vi "APT_Joystick.vi"() -> ()   [LabVIEW 2015]
uses:
  <vilib>/Utility/inputDevices.llb/joystickAcquire.vi
  Global Variable/GV_Lock State.vi
  Global Variable/GV_Z axis.vi
  <vilib>/Utility/inputDevices.llb/closeJoystick.vi
panel:
  out "Lock State":dbl=18.0
  out "lock":bool
  in  "error in (no error)":errorcluster caption="错误输入（无错误）"
  in  "MG17Motor Y":refnum<k7>(container)
  in  "选项卡控件":enum32{"APT Controller", "Parameters"}(tab)
  in  "Absolute y":dbl
  in  "Stop Device":bool
  in  "y Down":bool
  in  "y Up":bool
  out "y lock":bool
  out "x lock":bool
  in  "Joystick Onoff":bool=TRUE
  in  "HWSerialNum Y":i32=26000520
  in  "Stop":bool
  in  "Home X":bool
  in  "Rel. Pos X":dbl=0.01 min=-10.0 max=360.0 format="%.4f"
  in  "Deviece Joystick":i32=5
  out "Display X":dbl(knob)=6.2977495193481445 scale=0.0..25.0
  out "Initial X":bool=TRUE
  out "Initial Y":bool=TRUE
  out "Display Y":dbl(knob)=20.590396881103516 scale=0.0..25.0
  in  "Home Y":bool
  in  "Rel. Pos Y":dbl=0.01 min=-10.0 max=360.0 format="%.4f"
  in  "HWSerialNum X":i32=26000634
  in  "x Down":bool
  in  "x Up":bool
  in  "Absolute x":dbl
  out "操纵杆信息":T1(array[cluster])=[{"axes total"=5, "buttons total"=10, "pov total"=1, "device name"="Controller (XBOX One For Windows)"}, {"axes total"=1, "buttons total"=1, "pov total"=0, "device name"="USB Keyboard"}, {"axes total"=0, "buttons total"=3, "pov total"=0, "device name"="USB Keyboard"}, {"axes total"=0, "buttons total"=21, "pov total"=0, "device name"="USB Keyboard"}]
  out "X axis":i32=797
  out "Y axis":i32=796
  out "Z axis":i32
  out "Y axis rotation":i32=-1813
  out "Axis Info":T2={"X axis"=797, "Y axis"=796, "Z axis"=0, "X axis rotation"=1154, "Y axis rotation"=-1813, "Z axis rotation"=0, "U axis"=0, "V axis"=0}
  out "按键信息":T3
  in  "下限":dbl
  in  "上限":dbl=25.0
  out "方向信息":T4={"pov 1"=-1, "pov 2"=-1, "pov 3"=-1, "pov 4"=-1}
  in  "MG17Motor X":refnum<k7>(container)
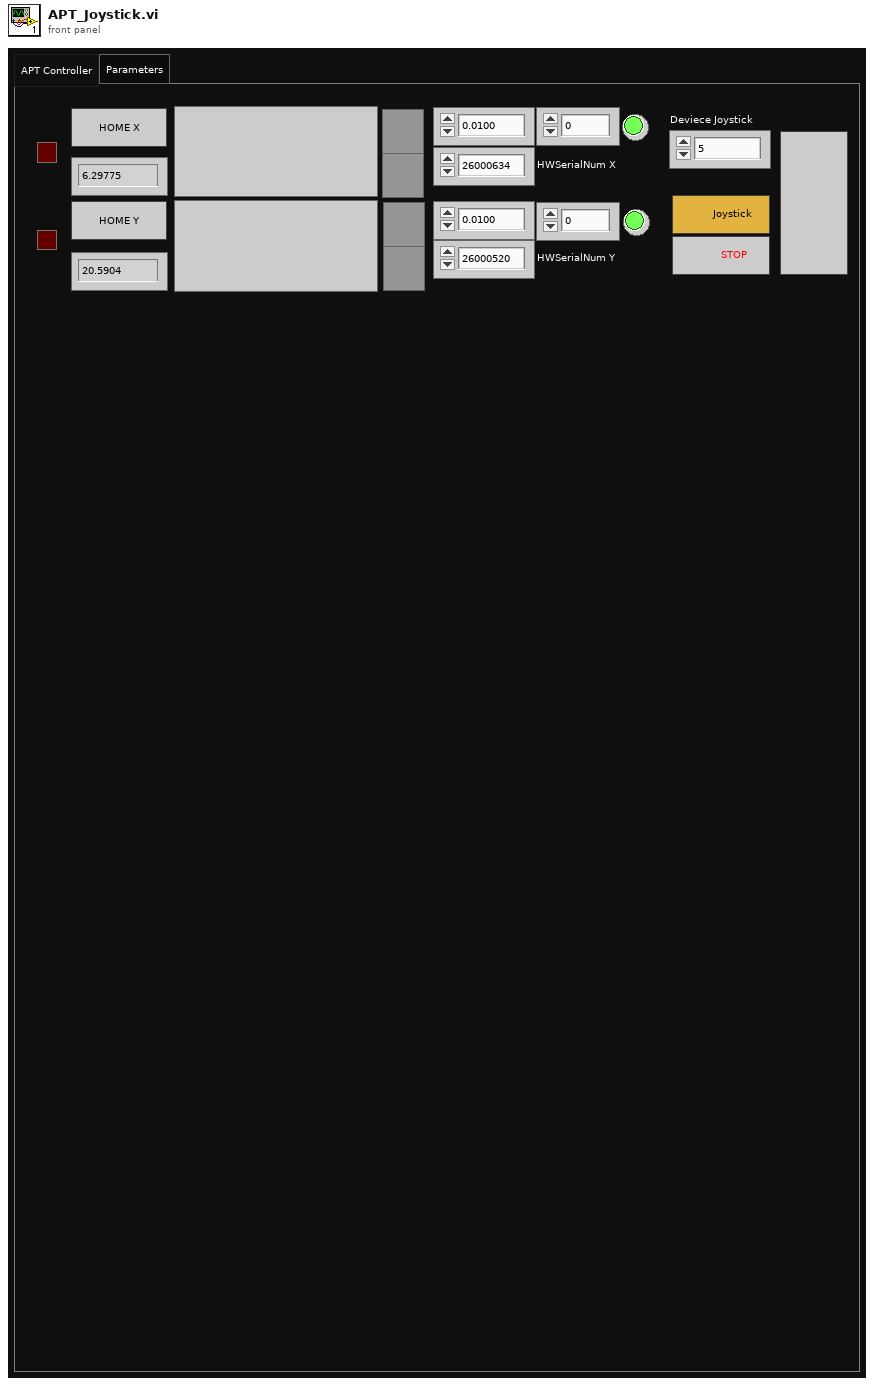
[diagram p1: front panel]
types:
  T1 = cluster{"axes total":u32, "buttons total":u32, "pov total":u32, "device name":string}[]
  T2 = cluster{"X axis":i32, "Y axis":i32, "Z axis":i32, "X axis rotation":i32, "Y axis rotation":i32, "Z axis rotation":i32, "U axis":i32, "V axis":i32}
  T3 = cluster{"button 1":bool, "button 2":bool, "button 3":bool, "button 4":bool, "button 5":bool, "button 6":bool, "button 7":bool, "button 8":bool, "button 9":bool, "button 10":bool, "button 11":bool, "button 12":bool, "button 13":bool, "button 14":bool, "button 15":bool, "button 16":bool, "button 17":bool, "button 18":bool, "button 19":bool, "button 20":bool, "button 21":bool, "button 22":bool, "button 23":bool, "button 24":bool, "button 25":bool, "button 26":bool, "button 27":bool, "button 28":bool, "button 29":bool, "button 30":bool, "button 31":bool, "button 32":bool}
  T4 = cluster{"pov 1":i32, "pov 2":i32, "pov 3":i32, "pov 4":i32}
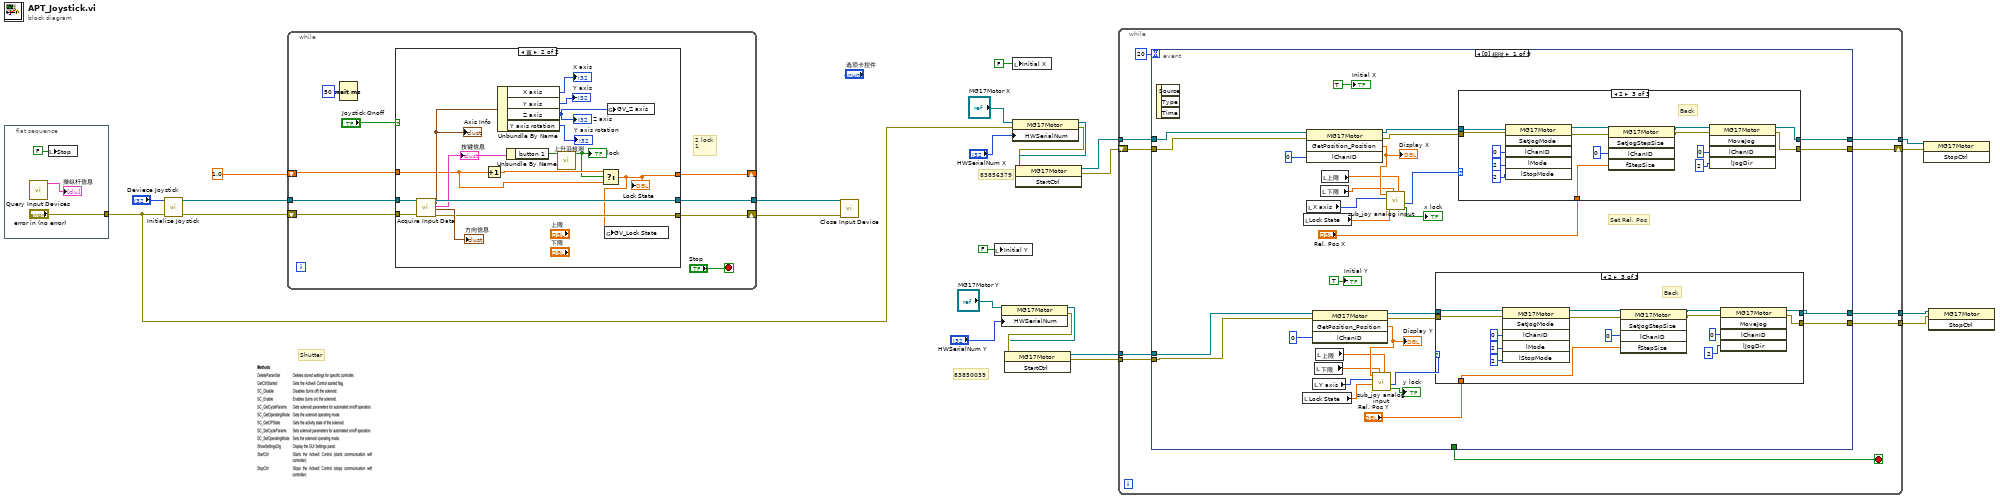
[diagram p0: block diagram]
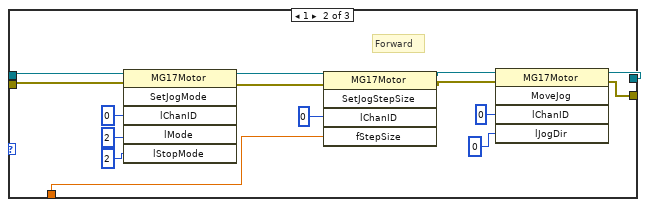
[diagram p3: hidden frame]
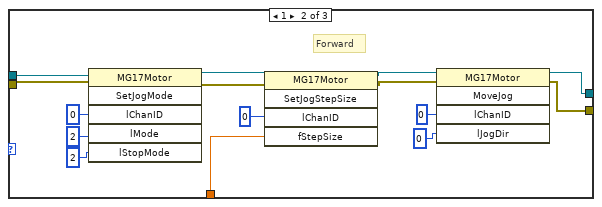
[diagram p5: hidden frame]
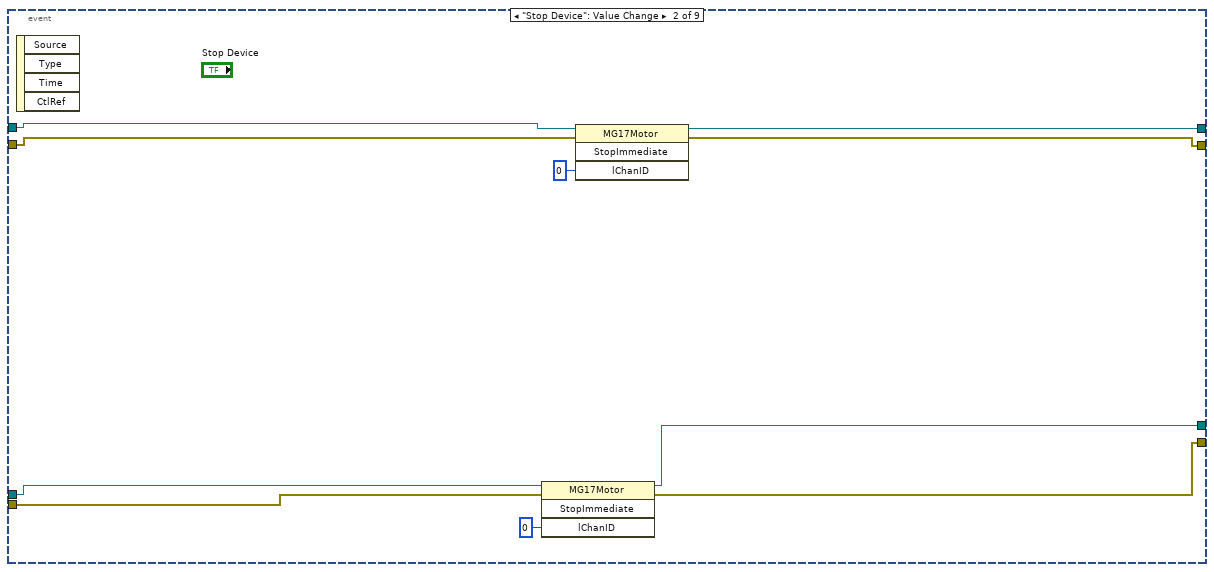
[diagram p6: hidden frame]
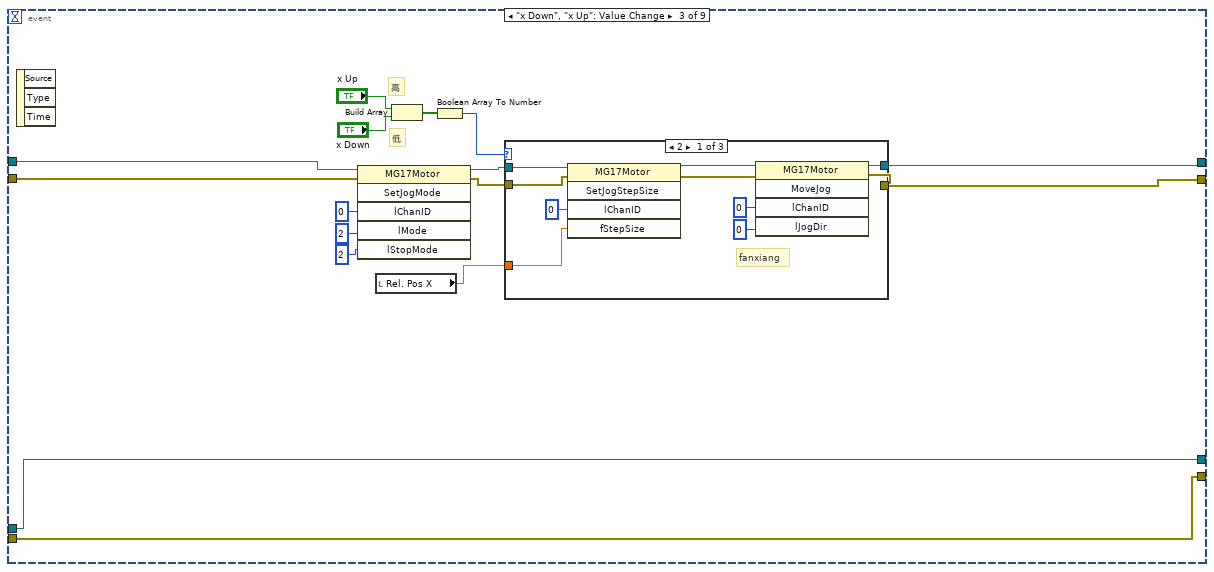
[diagram p7: hidden frame]
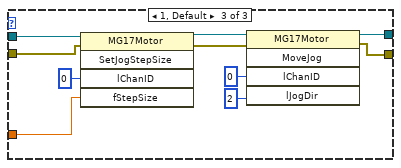
[diagram p9: hidden frame]
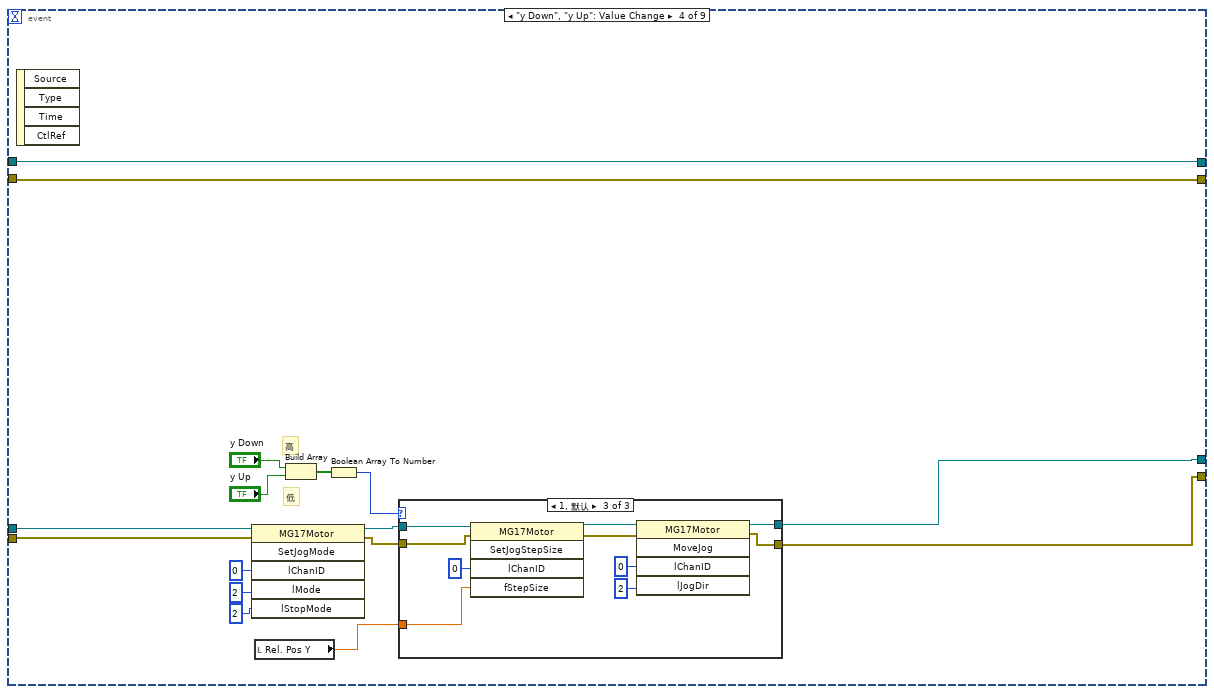
[diagram p10: hidden frame]
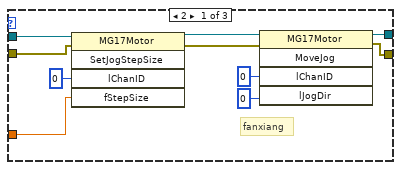
[diagram p11: hidden frame]
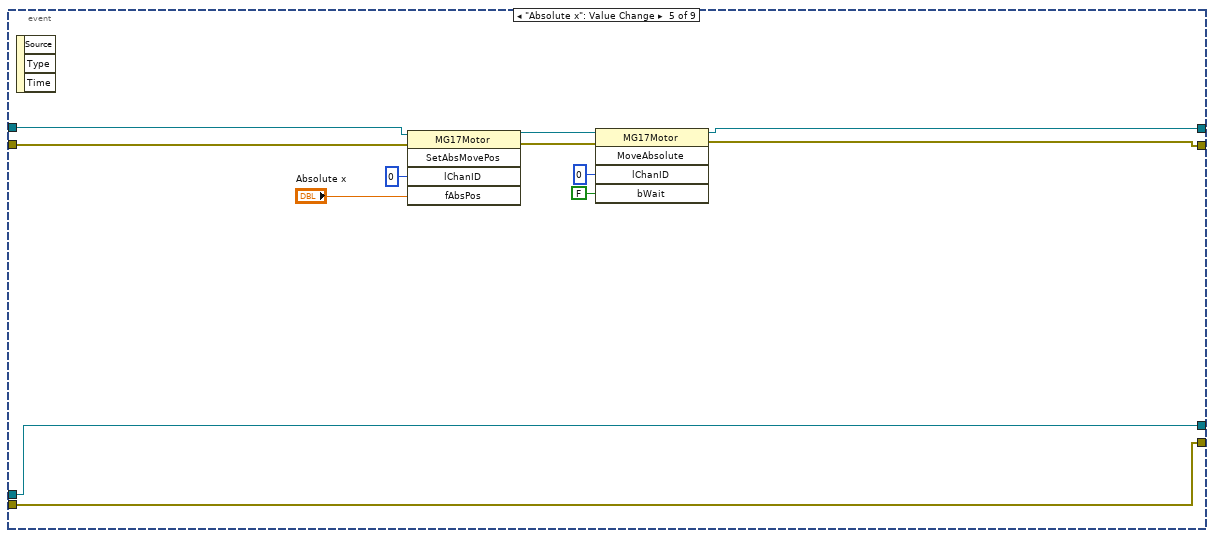
[diagram p13: hidden frame]
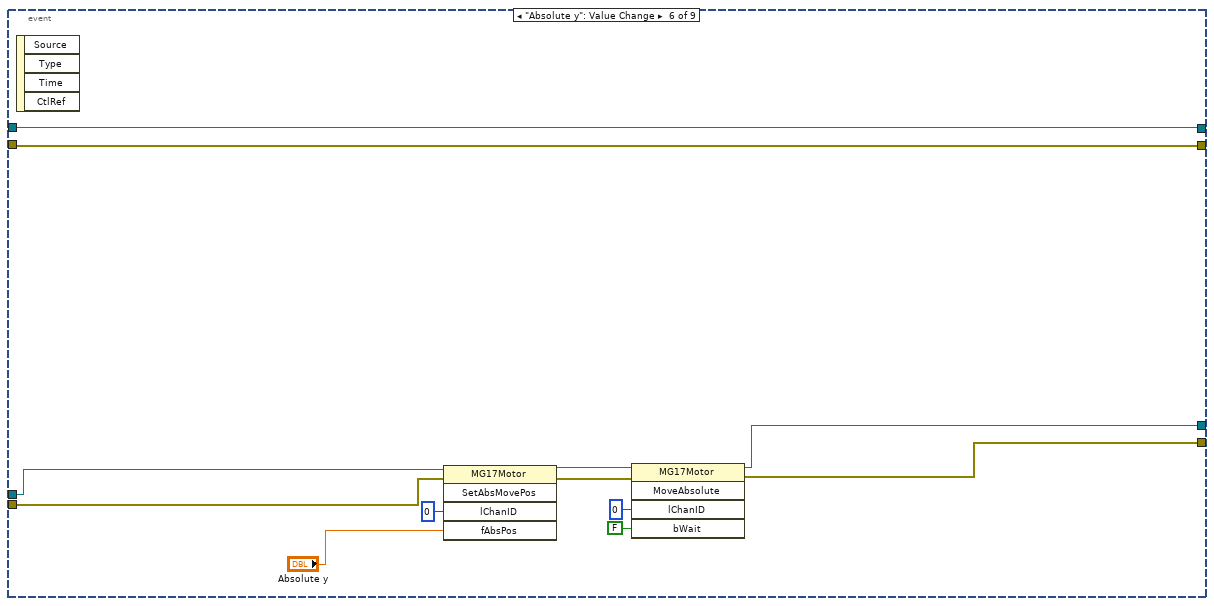
[diagram p14: hidden frame]
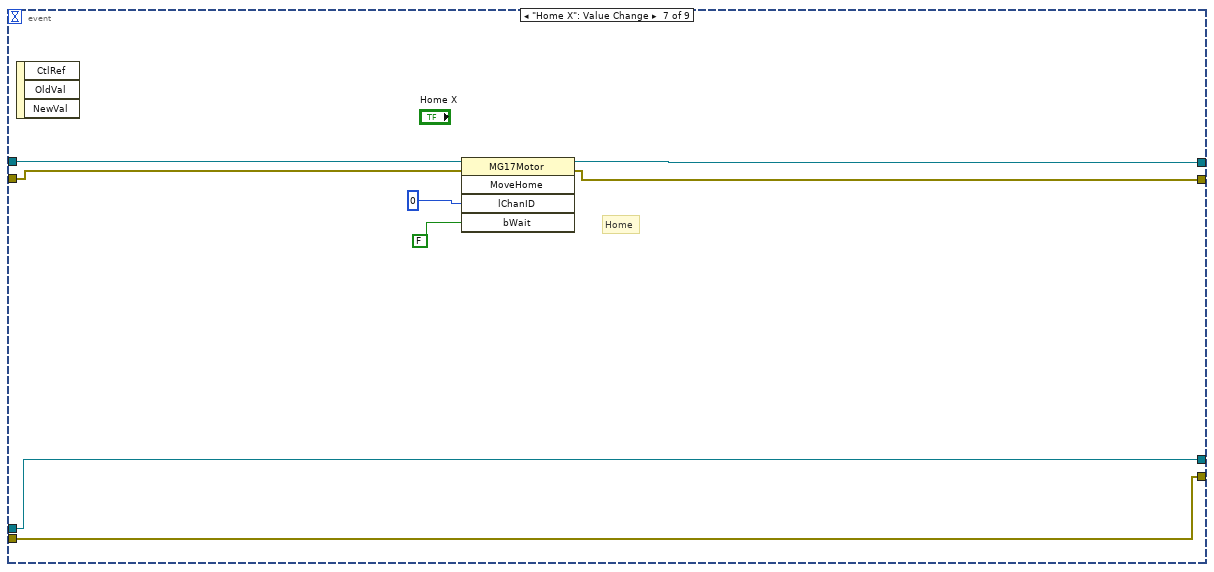
[diagram p15: hidden frame]
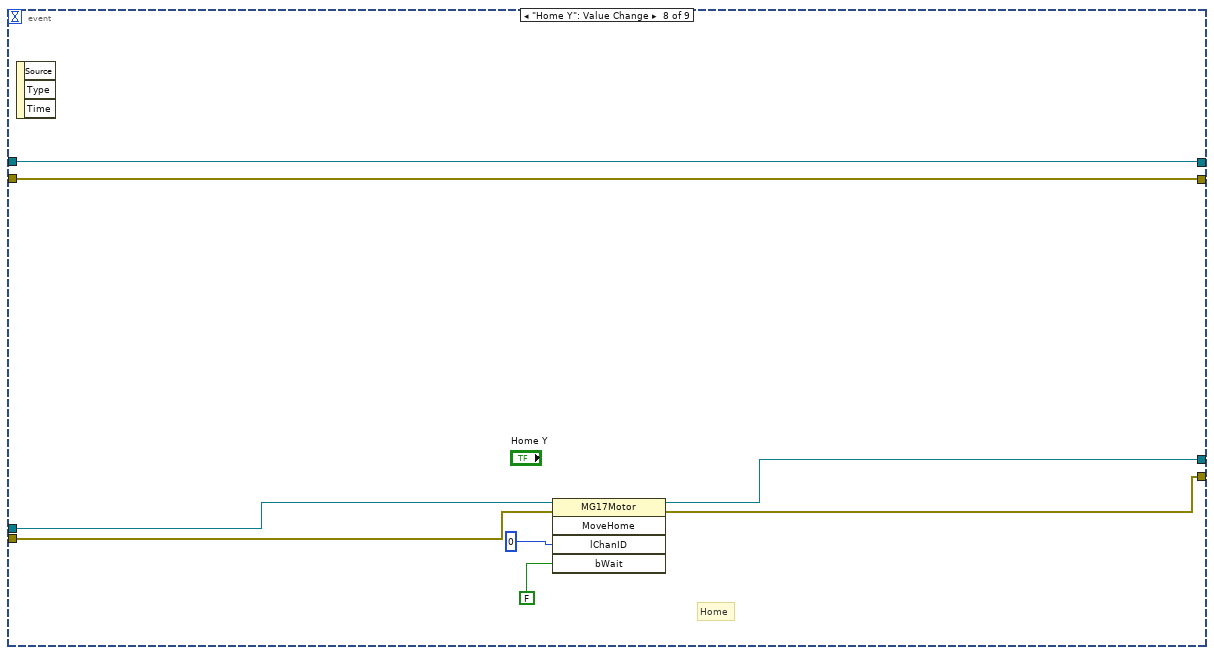
[diagram p16: hidden frame]
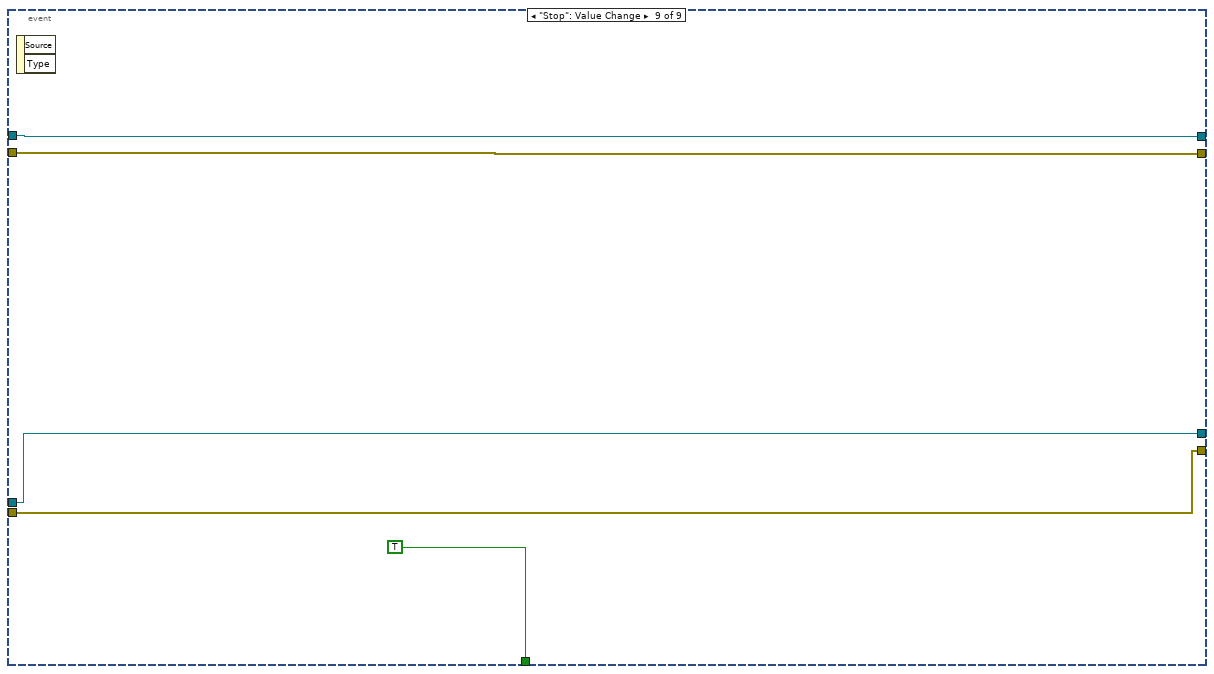
[diagram p17: hidden frame]
diagram:
  # "83856379"
  # "83850039"
  # "Shutter"
  n1 = flat-sequence {
    tunnel: ["error in (no error)"] -> w19
    frame #0 {
      n2 = call <vilib>:"Query Input Devices.vi"() -> ("joystick info"=→"操纵杆信息":T1)  [unwired: 8 in, 3 out]
      n3 = local write "Stop"(FALSE ("Stop")) -> ()
    }
  }
  n4 = call <vilib>:"Initialize Joystick.vi"("error in (no error)"=w19, "device index"="Deviece Joystick") -> ("error out"=w23:errorcluster, "device ID"=w24:refnum<k1>)  [unwired: 8 in]
  n5 = while {
    tunnel: w24 -> [w35]
    tunnel: [w33] -> w22
    shift-right: [w32] -> w21
    shift-left: w23 -> [w34]
    shift-right: [w29] -> _
    shift-left: 1.0 -> [w30]
    stop <- "Stop" stop-if-true
    # "2 lock\n1"
    n6 = Wait (ms)(milliseconds to wait=u32 50 ("等待时间（毫秒）")) -> ()  [unwired: 1 out]
    n7 = case shown="真" "Joystick Onoff" {
      tunnel: w35 -> [w40 w55]
      tunnel: w34 -> [w39 w54]
      tunnel: [w40 w53] -> w33
      tunnel: [w39 w52] -> w32
      tunnel: w30 -> [w38 w45]
      tunnel: [w38 w41] -> w29
      frame False {
      }
      frame True {
        n8 = call-poly <vilib>:"Acquire Input Data.vi"("device ID"=w55, "error in (no error)"=w54) -> ("device ID"=w53:refnum<k1>, "axis info"=w51:T2, "button info"=w47:T3, "direction info"=→"方向信息":T4, "error out"=w52:errorcluster)  [unwired: 13 in]
        "按键信息" <- w47
        "Axis Info" <- w51
        n9 = Increment(x=w45) -> (x+1=w46:dbl)
        n10 = Unbundle By Name(w51) -> ("X axis"=→"X axis":i32, "Y axis"=→"Y axis":i32, "Z axis"=w42:i32, "Y axis rotation"=→"Y axis rotation":i32)
        "Z axis" <- w42
        n11 = Unbundle By Name(w47) -> ("button 1"=w44:bool)
        n12 = call "上升沿检测.vi"("input"=w44) -> ("output"=w43:bool)  [unwired: 9 in, 1 out]
        "lock" <- w43
        n13 = Select(t=w46, s=w43, f=w45) -> (s? t:f=w41:dbl)
        "Lock State" <- w41
        n14 = global write "GV_Lock State.vi" "GV_Lock State"(w41) -> ()
        n15 = global write "GV_Z axis.vi" "GV_Z axis"(w42) -> ()
      }
    }
  }
  n16 = call-poly <vilib>:"Close Input Device.vi"("error in (no error)"=w21, "device ID"=w22) -> ()  [unwired: 8 in, 1 out]
  n17 = local write "Initial Y"(FALSE ("Initial")) -> ()
  n18 = property class="MG17Motor"(reference="MG17Motor Y", "HWSerialNum"="HWSerialNum Y") -> (reference out=w15:refnum<k7>, error out=w16:errorcluster)  [unwired: 1 in]
  n19 = invoke class="MG17Motor" method="StartCtrl"(reference=w15, error in=w16) -> (reference out=w4:refnum<k7>, error out=w3:errorcluster)  [unwired: 1 in, 1 out]
  n20 = property class="MG17Motor"(reference="MG17Motor X", error in=w19, "HWSerialNum"="HWSerialNum X") -> (reference out=w12:refnum<k7>, error out=w11:errorcluster)
  n21 = local write "Initial X"(FALSE ("Initial")) -> ()
  n22 = invoke class="MG17Motor" method="StartCtrl"(reference=w12, error in=w11) -> (reference out=w10:refnum<k7>, error out=w9:errorcluster)  [unwired: 1 in, 1 out]
  n23 = while {
    shift-right: [w63] -> w7
    shift-left: w9 -> [w65]
    tunnel: w10 -> [w66]
    tunnel: [w64] -> w8
    tunnel: w4 -> [w60]
    tunnel: w3 -> [w59]
    tunnel: [w58] -> w2
    tunnel: [w57] -> w1
    stop <- w61 stop-if-true
    n24 = event shown="[0] 超时" {
      selector: _ -> [_ _ _ _ _ _ _ _ _]
      dyn-events: _ -> [_ _ _ _ _ _ _ _ _]
      timeout: 20 -> [_ _ _ _ _ _ _ _ _]
      tunnel: w66 -> [w97 w166 w179 w212 w255 w262 w278 w282 w292]
      tunnel: w65 -> [w96 w165 w178 w211 w254 w261 w277 w281 w291]
      tunnel: [w92 w164 w177 w212 w253 w262 w276 w282 w292] -> w64
      tunnel: [w91 w163 w176 w211 w252 w261 w275 w281 w291] -> w63
      tunnel: [_ _ _ _ _ _ _ _ TRUE ("Stop")] -> w61
      tunnel: w60 -> [w70 w170 w174 w216 w250 w267 w274 w286 w290]
      tunnel: w59 -> [w69 w169 w173 w215 w249 w266 w273 w285 w289]
      tunnel: [w68 w168 w174 w214 w250 w265 w274 w284 w290] -> w58
      tunnel: [w67 w167 w173 w213 w249 w264 w273 w283 w289] -> w57
      event Timeout {
        # "Set Rel. Pos"
        n25 = event-data() -> ()  [unwired: 1 in, 3 out]
        n26 = local read "Lock State"() -> (w76:dbl)
        n27 = local read "Lock State"() -> (w87:dbl)
        n28 = invoke class="MG17Motor" method="GetPosition_Position"(reference=w97, error in=w96, "lChanID"=0) -> (reference out=w94:refnum<k7>, error out=w93:errorcluster, "GetPosition_Position"=w85:sgl)  [unwired: 1 in, 1 out]
        "Display X" <- w85
        n29 = local read "X axis"() -> (w86:i32)
        n30 = invoke class="MG17Motor" method="GetPosition_Position"(reference=w70, error in=w69, "lChanID"=0) -> (reference out=w80:refnum<k7>, error out=w79:errorcluster, "GetPosition_Position"=w73:sgl)  [unwired: 1 in, 1 out]
        "Display Y" <- w73
        n31 = local read "Y axis"() -> (w74:i32)
        n32 = local read "下限"() -> (w71:dbl)
        n33 = local read "上限"() -> (w72:dbl)
        n34 = local read "下限"() -> (w83:dbl)
        n35 = local read "上限"() -> (w84:dbl)
        n36 = call "sub_joy analog input.vi"("上限"=w72, "下限"=w71, "lock输入奇偶"=w76, "x"=w74, "Displacement"=w73) -> ("lock dis."=→"y lock":bool, "x state"=w77:i32)  [unwired: 5 in]
        n37 = call "sub_joy analog input.vi"("上限"=w84, "下限"=w83, "lock输入奇偶"=w87, "x"=w86, "Displacement"=w85) -> ("lock dis."=→"x lock":bool, "x state"=w90:i32)  [unwired: 5 in]
        n38 = case shown="2" w77 {
          tunnel: w80 -> [w100 w104 w119]
          tunnel: w79 -> [w99 w103 w118]
          tunnel: [w100 w111 w126] -> w68
          tunnel: [w99 w110 w125] -> w67
          tunnel: "Rel. Pos Y" -> [_ w109 w124]
          frame 0, Default {
          }
          frame 1 {
            # "Forward"
            n39 = invoke class="MG17Motor" method="SetJogMode"(reference=w104, error in=w103, "lChanID"=0, "lMode"=2, "lStopMode"=2) -> (reference out=w102:refnum<k7>, error out=w101:errorcluster)  [unwired: 1 in, 4 out]
            n40 = invoke class="MG17Motor" method="SetJogStepSize"(reference=w102, error in=w101, "lChanID"=0, "fStepSize"=w109) -> (reference out=w113:refnum<k7>, error out=w112:errorcluster)  [unwired: 1 in, 3 out]
            n41 = invoke class="MG17Motor" method="MoveJog"(reference=w113, error in=w112, "lChanID"=0, "lJogDir"=0) -> (reference out=w111:refnum<k7>, error out=w110:errorcluster)  [unwired: 1 in, 3 out]
          }
          frame 2 {
            # "Back"
            n42 = invoke class="MG17Motor" method="SetJogMode"(reference=w119, error in=w118, "lChanID"=0, "lMode"=2, "lStopMode"=2) -> (reference out=w117:refnum<k7>, error out=w116:errorcluster)  [unwired: 1 in, 4 out]
            n43 = invoke class="MG17Motor" method="SetJogStepSize"(reference=w117, error in=w116, "lChanID"=0, "fStepSize"=w124) -> (reference out=w128:refnum<k7>, error out=w127:errorcluster)  [unwired: 1 in, 3 out]
            n44 = invoke class="MG17Motor" method="MoveJog"(reference=w128, error in=w127, "lChanID"=0, "lJogDir"=2) -> (reference out=w126:refnum<k7>, error out=w125:errorcluster)  [unwired: 1 in, 3 out]
          }
        }
        n45 = case shown="2" w90 {
          tunnel: w94 -> [w132 w135 w150]
          tunnel: w93 -> [w131 w136 w151]
          tunnel: [w132 w143 w158] -> w92
          tunnel: [w131 w142 w157] -> w91
          tunnel: "Rel. Pos X" -> [_ w141 w156]
          frame 0, Default {
          }
          frame 1 {
            # "Forward"
            n46 = invoke class="MG17Motor" method="SetJogMode"(reference=w135, error in=w136, "lChanID"=0, "lMode"=2, "lStopMode"=2) -> (reference out=w134:refnum<k7>, error out=w133:errorcluster)  [unwired: 1 in, 4 out]
            n47 = invoke class="MG17Motor" method="SetJogStepSize"(reference=w134, error in=w133, "lChanID"=0, "fStepSize"=w141) -> (reference out=w145:refnum<k7>, error out=w144:errorcluster)  [unwired: 1 in, 3 out]
            n48 = invoke class="MG17Motor" method="MoveJog"(reference=w145, error in=w144, "lChanID"=0, "lJogDir"=0) -> (reference out=w143:refnum<k7>, error out=w142:errorcluster)  [unwired: 1 in, 3 out]
          }
          frame 2 {
            # "Back"
            n49 = invoke class="MG17Motor" method="SetJogMode"(reference=w150, error in=w151, "lChanID"=0, "lMode"=2, "lStopMode"=2) -> (reference out=w149:refnum<k7>, error out=w148:errorcluster)  [unwired: 1 in, 4 out]
            n50 = invoke class="MG17Motor" method="SetJogStepSize"(reference=w149, error in=w148, "lChanID"=0, "fStepSize"=w156) -> (reference out=w160:refnum<k7>, error out=w159:errorcluster)  [unwired: 1 in, 3 out]
            n51 = invoke class="MG17Motor" method="MoveJog"(reference=w160, error in=w159, "lChanID"=0, "lJogDir"=2) -> (reference out=w158:refnum<k7>, error out=w157:errorcluster)  [unwired: 1 in, 3 out]
          }
        }
        "Initial X" <- TRUE ("Initial")
        "Initial Y" <- TRUE ("Initial")
      }
      event "Stop Device": Value Change {
        n52 = event-data() -> ()  [unwired: 1 in, 4 out]
        n53 = invoke class="MG17Motor" method="StopImmediate"(reference=w170, error in=w169, "lChanID"=0) -> (reference out=w168:refnum<k7>, error out=w167:errorcluster)  [unwired: 1 in, 2 out]
        n54 = invoke class="MG17Motor" method="StopImmediate"(reference=w166, error in=w165, "lChanID"=0) -> (reference out=w164:refnum<k7>, error out=w163:errorcluster)  [unwired: 1 in, 2 out]
      }
      event "x Down", "x Up": Value Change {
        # "低"
        # "高"
        n55 = event-data() -> ()  [unwired: 1 in, 3 out]
        n56 = invoke class="MG17Motor" method="SetJogMode"(reference=w179, error in=w178, "lChanID"=0, "lMode"=2, "lStopMode"=2) -> (reference out=w184:refnum<k7>, error out=w185:errorcluster)  [unwired: 1 in, 4 out]
        n57 = local read "Rel. Pos X"() -> (w175:dbl)
        n58 = Build Array("x Up", "x Down") -> (w182:bool[])
        n59 = Boolean Array To Number(Boolean array=w182) -> (number=w183:u32)
        n60 = case shown="2" w183 {
          tunnel: w184 -> [w198 w200 w210]
          tunnel: [w196 w200 w208] -> w177
          tunnel: w185 -> [w193 w199 w205]
          tunnel: [w191 w199 w203] -> w176
          tunnel: w175 -> [w189 _ w201]
          frame 2 {
            # "fanxiang"
            n61 = invoke class="MG17Motor" method="SetJogStepSize"(reference=w198, error in=w193, "lChanID"=0, "fStepSize"=w189) -> (reference out=w197:refnum<k7>, error out=w192:errorcluster)  [unwired: 1 in, 3 out]
            n62 = invoke class="MG17Motor" method="MoveJog"(reference=w197, error in=w192, "lChanID"=0, "lJogDir"=0) -> (reference out=w196:refnum<k7>, error out=w191:errorcluster)  [unwired: 1 in, 3 out]
          }
          frame 0 {
          }
          frame 1, Default {
            n63 = invoke class="MG17Motor" method="SetJogStepSize"(reference=w210, error in=w205, "lChanID"=0, "fStepSize"=w201) -> (reference out=w209:refnum<k7>, error out=w204:errorcluster)  [unwired: 1 in, 3 out]
            n64 = invoke class="MG17Motor" method="MoveJog"(reference=w209, error in=w204, "lChanID"=0, "lJogDir"=2) -> (reference out=w208:refnum<k7>, error out=w203:errorcluster)  [unwired: 1 in, 3 out]
          }
        }
      }
      event "y Down", "y Up": Value Change {
        # "低"
        # "高"
        n65 = event-data() -> ()  [unwired: 1 in, 4 out]
        n66 = invoke class="MG17Motor" method="SetJogMode"(reference=w216, error in=w215, "lChanID"=0, "lMode"=2, "lStopMode"=2) -> (reference out=w222:refnum<k7>, error out=w223:errorcluster)  [unwired: 1 in, 4 out]
        n67 = local read "Rel. Pos Y"() -> (w217:dbl)
        n68 = Build Array("y Down", "y Up") -> (w220:bool[])
        n69 = Boolean Array To Number(Boolean array=w220) -> (number=w221:u32)
        n70 = case shown="1, 默认" w221 {
          tunnel: w222 -> [w236 w238 w248]
          tunnel: [w234 w238 w246] -> w214
          tunnel: w223 -> [w231 w237 w243]
          tunnel: [w229 w237 w241] -> w213
          tunnel: w217 -> [w227 _ w239]
          frame 2 {
            # "fanxiang"
            n71 = invoke class="MG17Motor" method="SetJogStepSize"(reference=w236, error in=w231, "lChanID"=0, "fStepSize"=w227) -> (reference out=w235:refnum<k7>, error out=w230:errorcluster)  [unwired: 1 in, 3 out]
            n72 = invoke class="MG17Motor" method="MoveJog"(reference=w235, error in=w230, "lChanID"=0, "lJogDir"=0) -> (reference out=w234:refnum<k7>, error out=w229:errorcluster)  [unwired: 1 in, 3 out]
          }
          frame 0 {
          }
          frame 1, Default {
            n73 = invoke class="MG17Motor" method="SetJogStepSize"(reference=w248, error in=w243, "lChanID"=0, "fStepSize"=w239) -> (reference out=w247:refnum<k7>, error out=w242:errorcluster)  [unwired: 1 in, 3 out]
            n74 = invoke class="MG17Motor" method="MoveJog"(reference=w247, error in=w242, "lChanID"=0, "lJogDir"=2) -> (reference out=w246:refnum<k7>, error out=w241:errorcluster)  [unwired: 1 in, 3 out]
          }
        }
      }
      event "Absolute x": Value Change {
        n75 = event-data() -> ()  [unwired: 1 in, 3 out]
        n76 = invoke class="MG17Motor" method="SetAbsMovePos"(reference=w255, error in=w254, "lChanID"=0, "fAbsPos"="Absolute x") -> (reference out=w260:refnum<k7>, error out=w257:errorcluster)  [unwired: 1 in, 3 out]
        n77 = invoke class="MG17Motor" method="MoveAbsolute"(reference=w260, error in=w257, "lChanID"=0, "bWait"=FALSE) -> (reference out=w253:refnum<k7>, error out=w252:errorcluster)  [unwired: 1 in, 3 out]
      }
      event "Absolute y": Value Change {
        n78 = event-data() -> ()  [unwired: 1 in, 4 out]
        n79 = invoke class="MG17Motor" method="SetAbsMovePos"(reference=w267, error in=w266, "lChanID"=0, "fAbsPos"="Absolute y") -> (reference out=w272:refnum<k7>, error out=w269:errorcluster)  [unwired: 1 in, 3 out]
        n80 = invoke class="MG17Motor" method="MoveAbsolute"(reference=w272, error in=w269, "lChanID"=0, "bWait"=FALSE) -> (reference out=w265:refnum<k7>, error out=w264:errorcluster)  [unwired: 1 in, 3 out]
      }
      event "Home X": Value Change {
        # "Home"
        n81 = event-data() -> ()  [unwired: 1 in, 3 out]
        n82 = invoke class="MG17Motor" method="MoveHome"(reference=w278, error in=w277, "lChanID"=0, "bWait"=FALSE) -> (reference out=w276:refnum<k7>, error out=w275:errorcluster)  [unwired: 1 in, 3 out]
      }
      event "Home Y": Value Change {
        # "Home"
        n83 = event-data() -> ()  [unwired: 1 in, 3 out]
        n84 = invoke class="MG17Motor" method="MoveHome"(reference=w286, error in=w285, "lChanID"=0, "bWait"=FALSE) -> (reference out=w284:refnum<k7>, error out=w283:errorcluster)  [unwired: 1 in, 3 out]
      }
      event "Stop": Value Change {
        n85 = event-data() -> ()  [unwired: 1 in, 2 out]
      }
    }
  }
  n86 = invoke class="MG17Motor" method="StopCtrl"(reference=w8, error in=w7) -> ()  [unwired: 1 in, 3 out]
  n87 = invoke class="MG17Motor" method="StopCtrl"(reference=w2, error in=w1) -> ()  [unwired: 1 in, 3 out]
